vi "RSNRPZ Get Scope Measurements Pulse Times.vi"(8 "error in (no error)":errorcluster, 10 "Channel (1)":i32=1, 11 "VISA session":refnum<visa-resource-name> caption="VISA resource name") -> (0 "error out":errorcluster, 1 "Duty Cycle":dbl format="%^.3e", 3 "dup VISA session":refnum<visa-resource-name> caption="VISA resource name", 4 "Pulse Duration":dbl format="%^.3e", 5 "Pulse Period":dbl format="%^.3e")   [LabVIEW 2010]
doc: "This VI returns the calculated pulse time parameters of the last recorded trace. If a parameter could not be calculated the returned value is NAN. The Sensor takes the time values when the trace crosses the reference level points for duration and period calculation.\n\nNote:\n1) This VI is only available for NRP-Z81.\n\nRemote-control command(s):\nSENS:TRAC:MEAS:PULS:DCYC?\nSENS:TRAC:MEAS:PULS:DUR?\nSENS:TRAC:MEAS:PULS:PER?"
uses:
  rsnrpz_32.dll
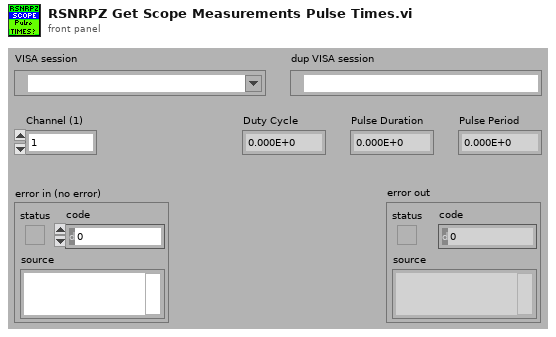
[diagram p1: front panel]
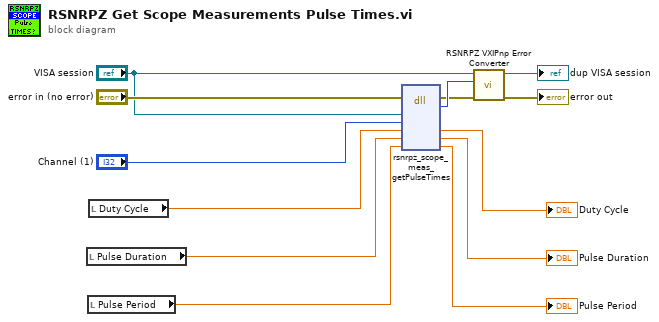
[diagram p0: block diagram]
diagram:
  n1 = local read "Pulse Duration"() -> (w9:dbl)
  n2 = local read "Pulse Period"() -> (w7:dbl)
  n3 = local read "Duty Cycle"() -> (w11:dbl)
  n4 = dll-call lib="rsnrpz_32.dll" fn="rsnrpz_scope_meas_getPulseTimes"(error in="error in (no error)", "Instrument Handle"="VISA session", "Channel"="Channel (1)", "Duty Cycle"=w11, "Pulse Duration"=w9, "Pulse Period"=w7) -> (error out=w5:errorcluster, "Status"=w13:i32, "Duty Cycle"=→"Duty Cycle":dbl, "Pulse Duration"=→"Pulse Duration":dbl, "Pulse Period"=→"Pulse Period":dbl)  [unwired: 4 in, 1 out]
  n5 = call <instrlib>:"RSNRPZ VXIPnp Error Converter.vi"("error in"=w5, "VXIPnp error code"=w13, "VISA session"="VISA session") -> ("error out"=→"error out":errorcluster, "dup VISA session"=→"dup VISA session":refnum<visa-resource-name>)  [unwired: 7 in]
